vi "Initialize.vi"(8 "error in (no error)":errorcluster, 9 "Device":string, 10 "VISA Com Port":refnum<visa-resource-name>, 11 "Simulado in":refnum<class "Simulado.lvclass">) -> (0 "error out":errorcluster, 3 "Simulado out":refnum<class "Simulado.lvclass">)   [LabVIEW 2020, in "Simulado.lvclass"]
uses:
  Simulado.lvclass
  Simulado.lvclass/Simulado.ctl
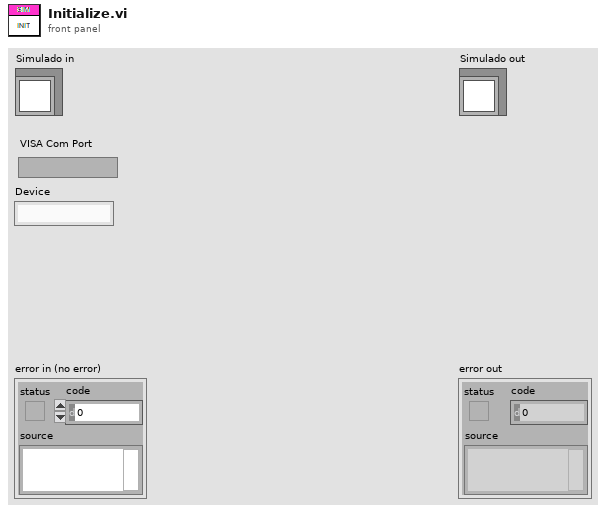
[diagram p1: front panel]
types:
  T1 = enum16{"Get Parameters", "Set Parameters", "Reset"}
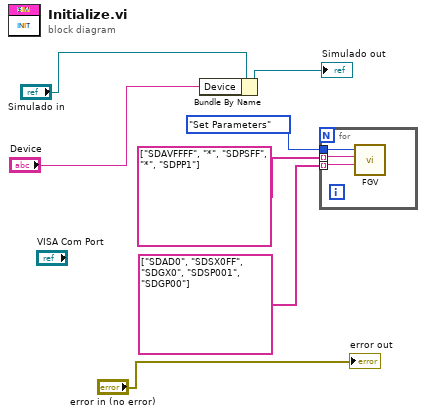
[diagram p0: block diagram]
diagram:
  n1 = Bundle By Name(cluster="Simulado in", "Device"="Device") -> (→"Simulado out":refnum<class "Simulado.lvclass">)
  n2 = for {
    tunnel: T1."Set Parameters" ("Función") -> [w10]
    tunnel: string[] ["SDAVFFFF", "*", "SDPSFF", "*", "SDPP1"] -> [w9] mode=indexing
    tunnel: string[] ["SDAD0", "SDSX0FF", "SDGX0", "SDSP001", "SDGP00"] -> [w8] mode=indexing
    n3 = call "FGV.vi"("Comandos"=w8, "Respuestas"=w9, "Función"=w10) -> ()  [unwired: 8 in, 1 out]
  }
  "error out" <- "error in (no error)"
